vi "create.vi"(6 "Exclude":bool, 7 "Actual":dbl, 8 "error in (no error)":errorcluster, 9 "Amount":dbl, 10 "Category Name":string, 11 "WhichMonth.lvclass":refnum<class "WhichMonth.lvclass">) -> (0 "error out":errorcluster, 3 "Outcome out":refnum<class "Outcome.lvclass">)   [LabVIEW 2018, in "Outcome.lvclass"]
uses:
  Outcome.lvclass
  WhichMonth/WhichMonth.lvclass
  Outcome.lvclass/Outcome.ctl
  Goal/Goal.lvclass
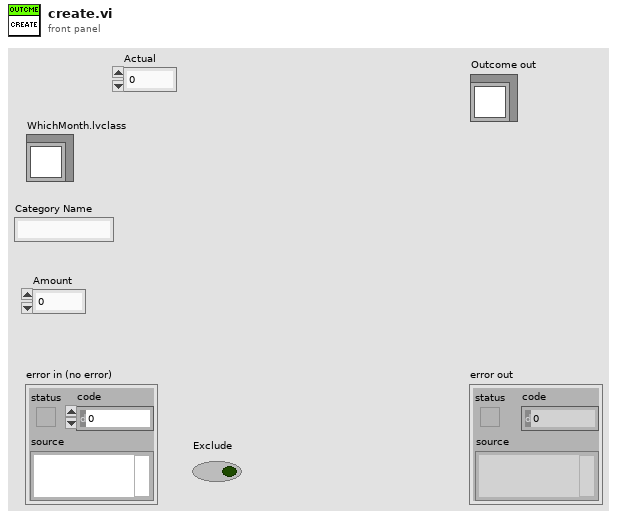
[diagram p1: front panel]
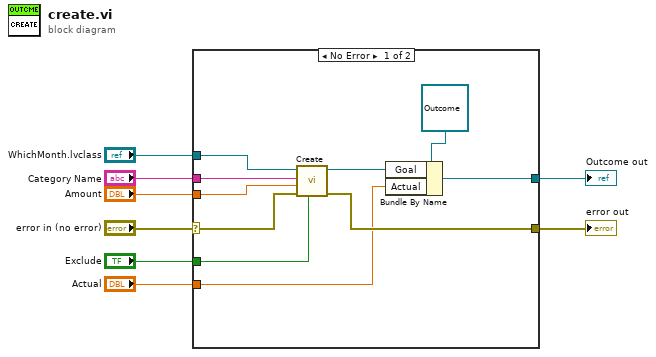
[diagram p0: block diagram]
diagram:
  n1 = case shown="No Error" "error in (no error)" {
    selector: "error in (no error)" -> [w14 w19]
    tunnel: [w15 w19] -> w7
    tunnel: [w17 _] -> w6
    tunnel: "WhichMonth.lvclass" -> [w13 _]
    tunnel: "Category Name" -> [w12 _]
    tunnel: "Amount" -> [w11 _]
    tunnel: "Actual" -> [w10 _]
    tunnel: "Exclude" -> [w9 _]
    frame No Error {
      n2 = call "Create.vi"("Exclude"=w9, "error in (no error)"=w14, "Amount"=w11, "Category Name"=w12, "WhichMonth.lvclass"=w13) -> ("error out"=w15:errorcluster, "Goal out"=w18:refnum<class "Goal.lvclass">)  [unwired: 5 in]
      n3 = Bundle By Name(cluster=refnum<class "Outcome.lvclass"> refnum ("Outcome in"), "Goal"=w18, "Actual"=w10) -> (w17:refnum<class "Outcome.lvclass">)
    }
    frame Error {
    }
  }
  "error out" <- w7
  "Outcome out" <- w6
